vi "Find Name List.vi"(1 "Bus Scan":T2[](array[typedef]) {"Status" format="%.0x"}, 2 "Instruments":T1[](array[typedef])) -> (0 "Names":string[](array[string]))   [LabVIEW 2020]
uses:
  Sub Controls/Instrument IDN.ctl
  Sub Controls/Instrument Match.ctl
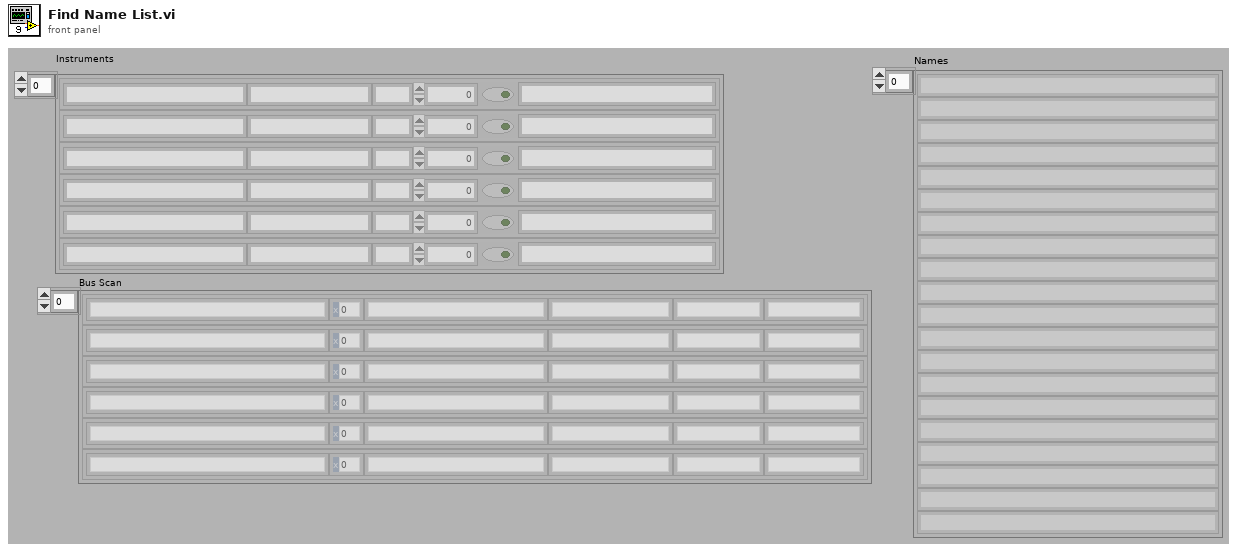
[diagram p1: front panel]
types:
  T1 = typedef "Instrument Match.ctl" = cluster{"Model":string, "Manufacturer":string, "Term Character":string, "Wait Time (mS)":u32, "Wait for SRQ":bool, "Type":string}
  T2 = typedef "Instrument IDN.ctl" = cluster{"VISA Address":string, "Status":u16, "Manufacturer":string, "Model":string, "Info":string, "Info 2":string, "Misc Data":variant}
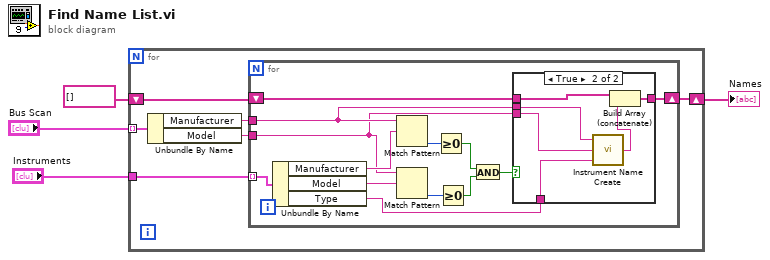
[diagram p0: block diagram]
diagram:
  n1 = for {
    tunnel: "Bus Scan" -> [w9] mode=indexing
    tunnel: "Instruments" -> [w10]
    shift-right: [w5] -> w2
    shift-left: string[] [] ("Names") -> [w6]
    n2 = Unbundle By Name(w9) -> ("Manufacturer"=w8:string, "Model"=w7:string)
    n3 = for {
      tunnel: w10 -> [w23] mode=indexing
      tunnel: w8 -> [w13]
      tunnel: w7 -> [w12]
      shift-right: [w14] -> w5
      shift-left: w6 -> [w15]
      n4 = Unbundle By Name(w23) -> ("Manufacturer"=w20:string, "Model"=w19:string, "Type"=w11:string)
      n5 = Match Pattern(string=w13, regular expression=w20) -> (offset past match=w22:i32)  [unwired: 1 in, 3 out]
      n6 = Match Pattern(string=w12, regular expression=w19) -> (offset past match=w21:i32)  [unwired: 1 in, 3 out]
      n7 = Greater Or Equal To 0?(x=w22) -> (x >= 0?=w17:bool)
      n8 = Greater Or Equal To 0?(x=w21) -> (x >= 0?=w18:bool)
      n9 = And(x=w17, y=w18) -> (x .and. y?=w16:bool)
      n10 = case shown="True" w16 {
        tunnel: w15 -> [w24 w29]
        tunnel: [w24 w30] -> w14
        tunnel: w13 -> [_ w27]
        tunnel: w12 -> [_ w28]
        tunnel: w11 -> [_ w25]
        frame False {
        }
        frame True {
          n11 = call "Instrument Name Create.vi"("Instrument Type"=w25, "Model"=w28, "Manufacturer"=w27) -> ("Name"=w26:string)
          n12 = Build Array (concatenate)(w29, w26) -> (w30:string[])
        }
      }
    }
  }
  "Names" <- w2
